vi "DataDisplaySubVi.vi"(5 "End":dbl, 7 "Start":dbl, 8 "10/20":bool, 9 "Reference":dbl, 10 "Data Display":dbl[][](array[numeric]), 11 "Data Cluster":T1) -> (2 "Data display(transposed)":dbl[][](array[numeric]), 3 "Data display":dbl[][](array[numeric]))   [LabVIEW 2020]
uses:
  controls/UI Data.ctl
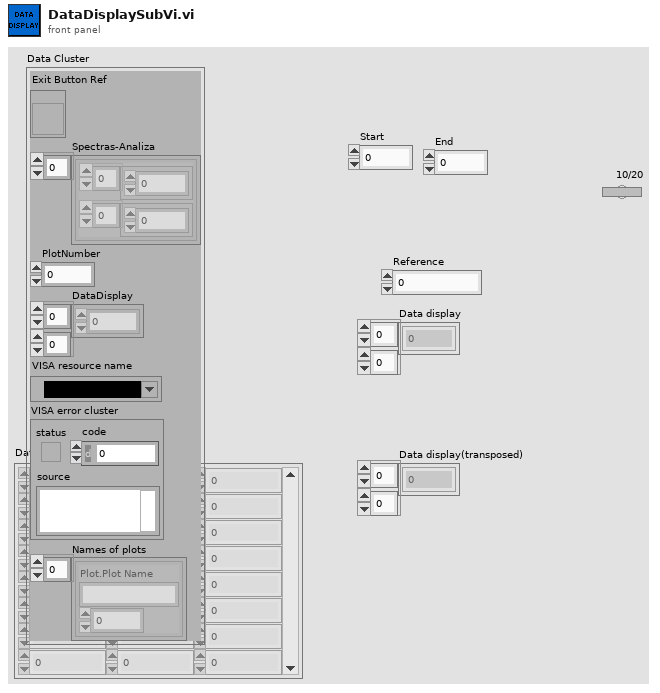
[diagram p1: front panel]
types:
  T1 = typedef "UI Data.ctl" = cluster{"Exit Button Ref":refnum<vi>, "Spectras-Analiza":cluster{dbl[], dbl[]}[], "PlotNumber":dbl, "DataDisplay":dbl[][], "VISA resource name":refnum<visa-resource-name>, "VISA error cluster":errorcluster, "Names of plots":cluster{"Plot.Plot Name":string, i32}[]}
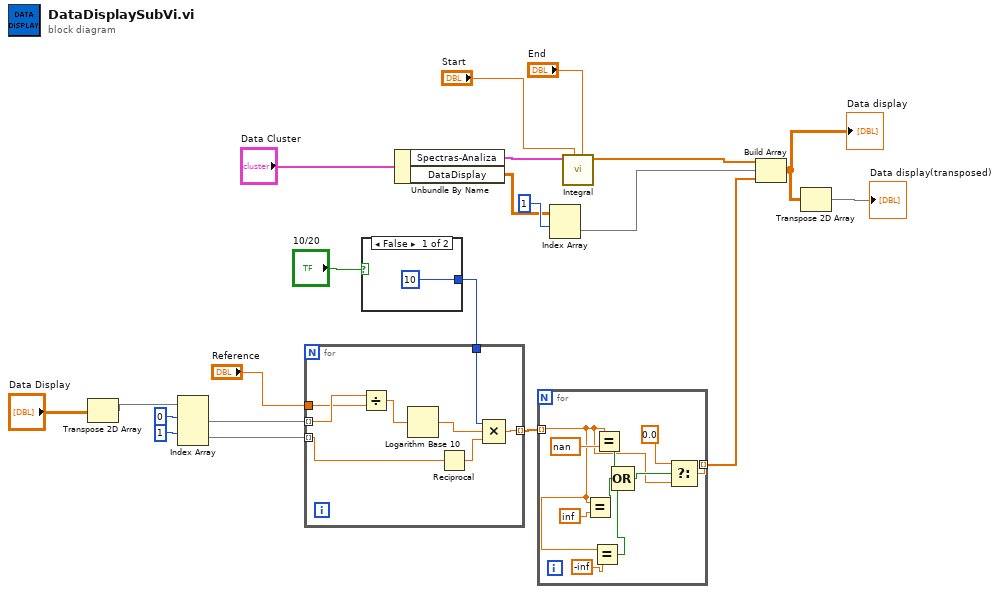
[diagram p0: block diagram]
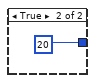
[diagram p2: hidden frame]
diagram:
  n1 = Transpose 2D Array(2D array="Data Display") -> (transposed array=w21:dbl[][])
  n2 = Index Array(array=w21, index (row) #1=0 ("index (row)"), index (row) #2=1 ("index (row)")) -> (element #1=w6:dbl[], element #2=w8:dbl[])  [unwired: 2 in]
  n3 = case shown="False" "10/20" {
    tunnel: [10 20] -> w1
    frame False {
    }
    frame True {
    }
  }
  n4 = for {
    tunnel: w8 -> [w31] mode=indexing
    tunnel: [w28] -> w7 mode=indexing
    tunnel: w6 -> [w26] mode=indexing
    tunnel: "Reference" -> [w25]
    tunnel: w1 -> [w24]
    n5 = Divide(x=w26, y=w25) -> (x/y=w27:dbl)
    n6 = Logarithm Base 10(1:w27) -> (0:w30:dbl)
    n7 = Reciprocal(x=w31) -> (1/x=w29:dbl)
    n8 = Compound Arithmetic op=MULTIPLY(w24, w30, w29) -> (w28:dbl)
  }
  n9 = Unbundle By Name("Data Cluster") -> ("Spectras-Analiza"=w10:cluster{dbl[], dbl[]}[], "DataDisplay"=w14:dbl[][])
  n10 = for {
    tunnel: w7 -> [w34] mode=indexing
    tunnel: [w39] -> w9 mode=indexing
    n11 = Equal?(x=w34, y=inf) -> (x = y?=w35:bool)
    n12 = Equal?(x=w34, y=-inf) -> (x = y?=w32:bool)
    n13 = Equal?(x=w34, y=nan) -> (x = y?=w37:bool)
    n14 = Compound Arithmetic op=OR(w37, w35, w32) -> (w38:bool)
    n15 = Select(t=0.0, s=w38, f=w34) -> (s? t:f=w39:dbl)
  }
  n16 = Index Array(array=w14, index (row)=1) -> (element=w16:dbl[])  [unwired: 1 in]
  n17 = call "Integral.vi"("End"="End", "Start"="Start", "Spectras-Analiza"=w10) -> ("Integral"=w11:dbl[])  [unwired: 8 in]
  n18 = Build Array(w11, w16, w9) -> (w18:dbl[][])
  "Data display" <- w18
  n19 = Transpose 2D Array(2D array=w18) -> (transposed array=→"Data display(transposed)":dbl[][])
